vi "Substitute Actor.vi"(10 "Substitute Actor in":refnum<class "Actor.lvclass">, 11 "Current Door Controller":refnum<class "Door Controller.lvclass">) -> (0 "error out":errorcluster, 2 "Substitute Actor out":refnum<class "Actor.lvclass">)   [LabVIEW 2020, in "Door Controller.lvlib" / "Door Controller.lvclass"]
doc: "(<B>Filename</B>: Actor Framework.lvlib:Actor.lvclass:Substitute Actor.vi)\n\nThis method copies information from the <b>Current Actor</b> to the <b>Substitute Actor</b>, including the to-self and the to-caller queue references. The purpose of this function is to allow an actor to define a method that replaces itself with another actor, useful for implementing a State Pattern Actor. Child classes should override this method to copy any additional fields that they need from the current to the substitute.\n\nThis method may return error code 678010: Illegal substitution. Overrides of this method may choose to return this error if the new actor is not one that is an appropriate substitute for the current actor, for whatever standards of \"appropriate\" are chosen for the current actor. If returning an error, override VIs should return the unmodified <b>Current Actor</b> as <b>Substitute Actor out</b>."
uses:
  Door Controller.lvclass
  C:/Program Files/National Instruments/LabVIEW 2020/vi.lib/ActorFramework/Actor/Actor.lvclass
  <vilib>/ActorFramework/Actor/Actor.lvclass
  Door Controller.lvclass/Door Controller.ctl
  Application/Application/Application.lvclass
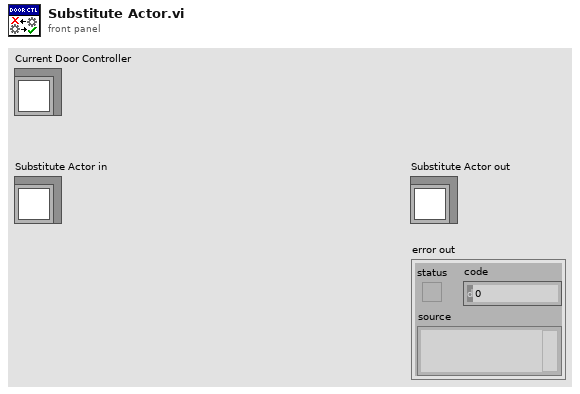
[diagram p1: front panel]
types:
  T1 = typedef "Door Interlocks.lvclass/Interlock Values.ctl" = cluster{"Door Open":bool, "Door Closed":bool, "Mode of Operation":T2}
  T2 = typedef "Door Interlocks.lvclass/Mode of Operation.ctl" = enum16{"Standard", "Interlock Override"}
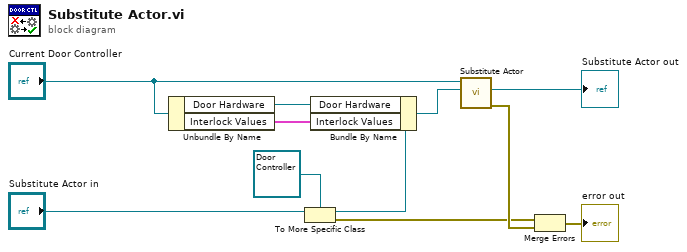
[diagram p0: block diagram]
diagram:
  n1 = Unbundle By Name("Current Door Controller") -> ("Door Hardware"=w5:refnum<class "Message Enqueuer.lvclass">, "Interlock Values"=w4:T1)
  n2 = To More Specific Class(target class=refnum<class "Door Controller.lvclass"> refnum ("Current Door Controller 2"), reference="Substitute Actor in") -> (specific class reference=w6:refnum<class "Door Controller.lvclass">, error out=w1:errorcluster)  [unwired: 1 in]
  n3 = Bundle By Name(cluster=w6, "Door Hardware"=w5, "Interlock Values"=w4) -> (w3:refnum<class "Door Controller.lvclass">)
  n4 = call-parent "Substitute Actor.vi"("Substitute Actor in"=w3, "Current Actor"="Current Door Controller") -> ("error out"=w11:errorcluster, "Substitute Actor out"=→"Substitute Actor out":refnum<class "Actor.lvclass">)  [unwired: 8 in]
  n5 = Merge Errors(w1, w11) -> (→"error out":errorcluster)
